vi "VBAI Initialize.vi"(8 "error in":errorcluster, 11 "File Name":string="Surface defect identify_1.vbai") -> (0 "error out":errorcluster, 3 "VBAI":cluster{"New Image":T1, "VBAI Session Out":T2})   [LabVIEW 2018]
uses:
  <vilib>/vision/Image Controls.llb/IMAQ Image.ctl
  <vilib>/userdefined/High Color/VBAIInterface.ctl
  <vilib>/vision/Vision Builder AI/API.llb/IVB Interface - VBAI Version.ctl
panel:
  out "Path":path=path "C:/Project/pk4soldering_v4.vbai"
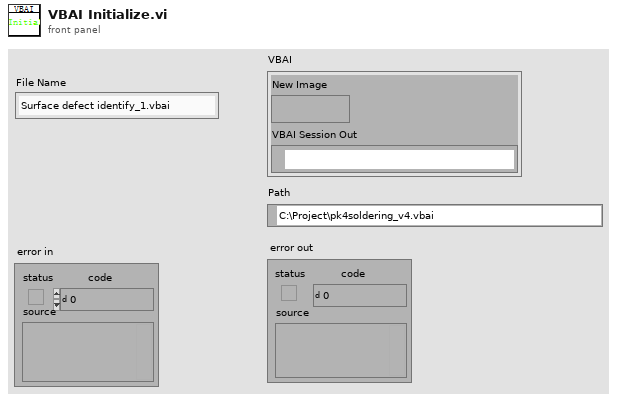
[diagram p1: front panel]
types:
  T1 = typedef "IMAQ Image.ctl" = refnum<image>
  T2 = typedef "VBAIInterface.ctl" = refnum<k21>
  T3 = typedef "IVB Interface - VBAI Version.ctl" = u16
  T4 = typedef "Image Type" = u32
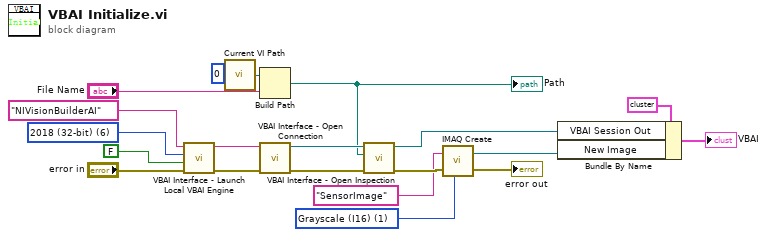
[diagram p0: block diagram]
diagram:
  w5 = T3 6 items=["2010 (32-bit)"=0, "2011 (32-bit)"=1, "2012 (32-bit)"=2, "2013 (32-bit)"=3, "2014 (32-bit)"=4, "2014 (64-bit)"=1004, "2015 (32-bit)"=5, "2015 (64-bit)"=1005, "2018 (32-bit)"=6, "2018 (64-bit)"=1006] ("Engine Version")
  w10 = T4 1 items=["Grayscale (U8)", "Grayscale (I16)", "Grayscale (SGL)", "Complex (CSG)", "RGB (U32)", "HSL (U32)", "RGB (U64)", "Grayscale (U16)"] ("Image Type")
  n1 = call <vilib>:"VBAI Interface - Launch Local VBAI Engine.vi"("error in"="error in", "Show VBAI Engine (True)"=FALSE, "Engine Version"=w5, "Local VBAI Engine Name"="NIVisionBuilderAI") -> ("error out"=w19:errorcluster, "Session Name Out"=w20:string)  [unwired: 6 in]
  n2 = call "Current VI Path.vi"("Time"=0) -> ("VI path"=w6:path)
  n3 = Build Path(base path=w6, name or relative path="File Name") -> (appended path=w11:path)
  "Path" <- w11
  n4 = call <vilib>:"VBAI Interface - Open Connection.vi"("error in"=w19, "Session In"=w20) -> ("error out"=w14:errorcluster, "Session Out"=w15:T2)  [unwired: 8 in]
  n5 = call <vilib>:"VBAI Interface - Open Inspection.vi"("error in"=w14, "Path"=w11, "Session In"=w15) -> ("error out"=w9:errorcluster, "Session Out"=w3:T2)  [unwired: 7 in]
  n6 = call "IMAQ Create"("Image Name"="SensorImage", "Image Type"=w10, "error in (no error)"=w9) -> ("New Image"=w2:T1, "error out"=→"error out":errorcluster)  [unwired: 2 in]
  n7 = Bundle By Name(cluster=cluster{"New Image":T1, "VBAI Session Out":T2} {"New Image"=refnum, "VBAI Session Out"=""} ("VBAI"), "VBAI Session Out"=w3, "New Image"=w2) -> (→"VBAI":cluster{"New Image":T1, "VBAI Session Out":T2})
